vi "PAN_FindCmdSetPath.vi"(10 "cmdset name":string) -> (2 "path":path)   [LabVIEW 2016]
uses:
  Modules/DBSHAND/private/vis/DatabaseHand_Element_Get(path).vi
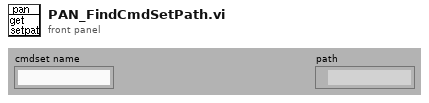
[diagram p1: front panel]
types:
  T1 = typedef "DatabaseHand_RefNum.ctl" = refnum<vi>
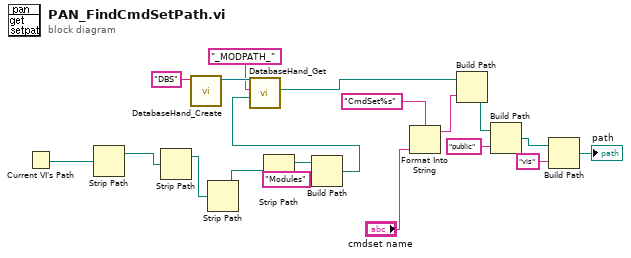
[diagram p0: block diagram]
diagram:
  n1 = Current VI's Path() -> (path=w19:path)
  n2 = Strip Path(path=w19) -> (stripped path=w15:path)  [unwired: 1 out]
  n3 = Strip Path(path=w15) -> (stripped path=w14:path)  [unwired: 1 out]
  n4 = call "DatabaseHand_Create.vi"("Name"="DBS") -> ("Database RefNum out"=w18:T1)  [unwired: 1 in, 9 out]
  n5 = Strip Path(path=w14) -> (stripped path=w13:path)  [unwired: 1 out]
  n6 = Strip Path(path=w13) -> (stripped path=w12:path)  [unwired: 1 out]
  n7 = Build Path(base path=w12, name or relative path="Modules") -> (appended path=w10:path)
  n8 = call-poly "DatabaseHand_Get.vi"("default value"=w10, "name"="_MODPATH_" ("group"), "Database RefNum in"=w18) -> ("value"=w9:path)  [unwired: 2 in, 6 out]
  n9 = Format Into String(format string="CmdSet%s", "cmdset name") -> (resulting string=w7:string)  [unwired: 2 in, 1 out]
  n10 = Build Path(base path=w9, name or relative path=w7) -> (appended path=w6:path)
  n11 = Build Path(base path=w6, name or relative path="public") -> (appended path=w4:path)
  n12 = Build Path(base path=w4, name or relative path="vis") -> (appended path=→"path":path)
